vi "Test.vi"(10 "Test Controls":T8 {"Belts" scale=-1.0..1.0; "Arm" scale=-1.0..1.0; "Drive Train" scale=-1.0..1.0}, 11 "Call Context":T16) -> (0 "Loop 2 Data":T12, 1 "SubState 2":T11, 2 "Loop 1 Data":T13, 3 "SubState 1":T11, 4 "SubState 3":T11, 5 "Loop 0 Data":T14, 6 "Loop 3 Data":T10, 7 "SubState 0":T11=enum."driver control", 8 "SubState 4":T15, 9 "Test Data":T9)   [LabVIEW 2013]
uses:
  typedefs/State Machine/subStates.ctl
  <vilib>/Rock Robotics/WPI/DriverStation/WPI_DriverStationDerivedRobotMode.ctl
  typedefs/State Machine/singleUseSubstate.ctl
  typedefs/Loop Datatypes/Loop 0 Datatype.ctl
  typedefs/Loop Datatypes/Loop 1 Datatype.ctl
  typedefs/Loop Datatypes/Loop 2 Datatype.ctl
  typedefs/Loop Datatypes/Loop 3 Datatype.ctl
  typedefs/Test/test data.ctl
  typedefs/Test/test controls.ctl
  <vilib>/Rock Robotics/WPI/Compressor/WPI_CompressorDevRef.ctl
  <vilib>/Rock Robotics/WPI/DigitalInput/WPI_DigitalInputDevRef.ctl
  <vilib>/Rock Robotics/SystemInterfaces/DIO/FPGA_DIOChannel.ctl
  <vilib>/Rock Robotics/SystemInterfaces/Typedef/FPGA_TypedefDigitalModule.ctl
  <vilib>/Rock Robotics/WPI/Relay/WPI_RelayDevRef.ctl
  <vilib>/Rock Robotics/SystemInterfaces/DIO/FPGA_DIORelayChannel.ctl
  <vilib>/Rock Robotics/WPI/Relay/WPI_RelayDirection.ctl
  typedefs/fg_typedef.ctl
  typedefs/DevRef Type.ctl
  <vilib>/Rock Robotics/WPI/Solenoid/WPI_SolenoidGetEnum.vi
  <vilib>/Rock Robotics/WPI/Joystick/WPI_JoystickGetSetRefNum.vi
  <vilib>/Rock Robotics/WPI/Compressor/WPI_CompressorGetSetRefNum.vi
panel:
  out "CompressorDevRef":T1={"DevStatus"={"status"=FALSE, "code"=0, "source"=""}, "DigitalInputDevRef"={"DevStatus"={"status"=FALSE, "code"=0, "source"=""}, "DIO Channel"=enum."DIO 1", "Digital Module"=enum."Digital Module 1"}, "RelayDevRef"={"DevStatus"={"status"=FALSE, "code"=0, "source"=""}, "Relay Channel"=enum."Invalid", "Digital Module"=enum."Digital Module 1", "Relay Direction"=enum."Both directions"}}
  out "Compressor":bool
  out "JS Axis-Y 3":dbl
  out "JS Axis-X 3":dbl
  out "JS Axis-Y 2":dbl
  out "JS Axis-X 2":dbl
  out "UDB":bool
  out "JS Axis-X":dbl
  out "JS Axis-Y":dbl
  out "Exit Value":i32=-1
  # "Loop Data and Substates"
  # "Drive Loop"
  # "State Machine Master Loop"
  # "Pickup/Passing Belts Loop"
  # "Pickup/Passing Arm Loop"
  # "Pneumatics Loop"
  # "Test Code (Only Run in \nTest Mode)"
  # "Pneumatics"
  # "Home Encoders"
  # "Manual Override"
  # "Joystick Control"
  # "Arm Safeties"
  # "Drive Safeties"
  # "Sensors"
  # "Drive Encoders"
  # "Pneumatics Commands"
  # "Compressor"
  # "Arm Encoder"
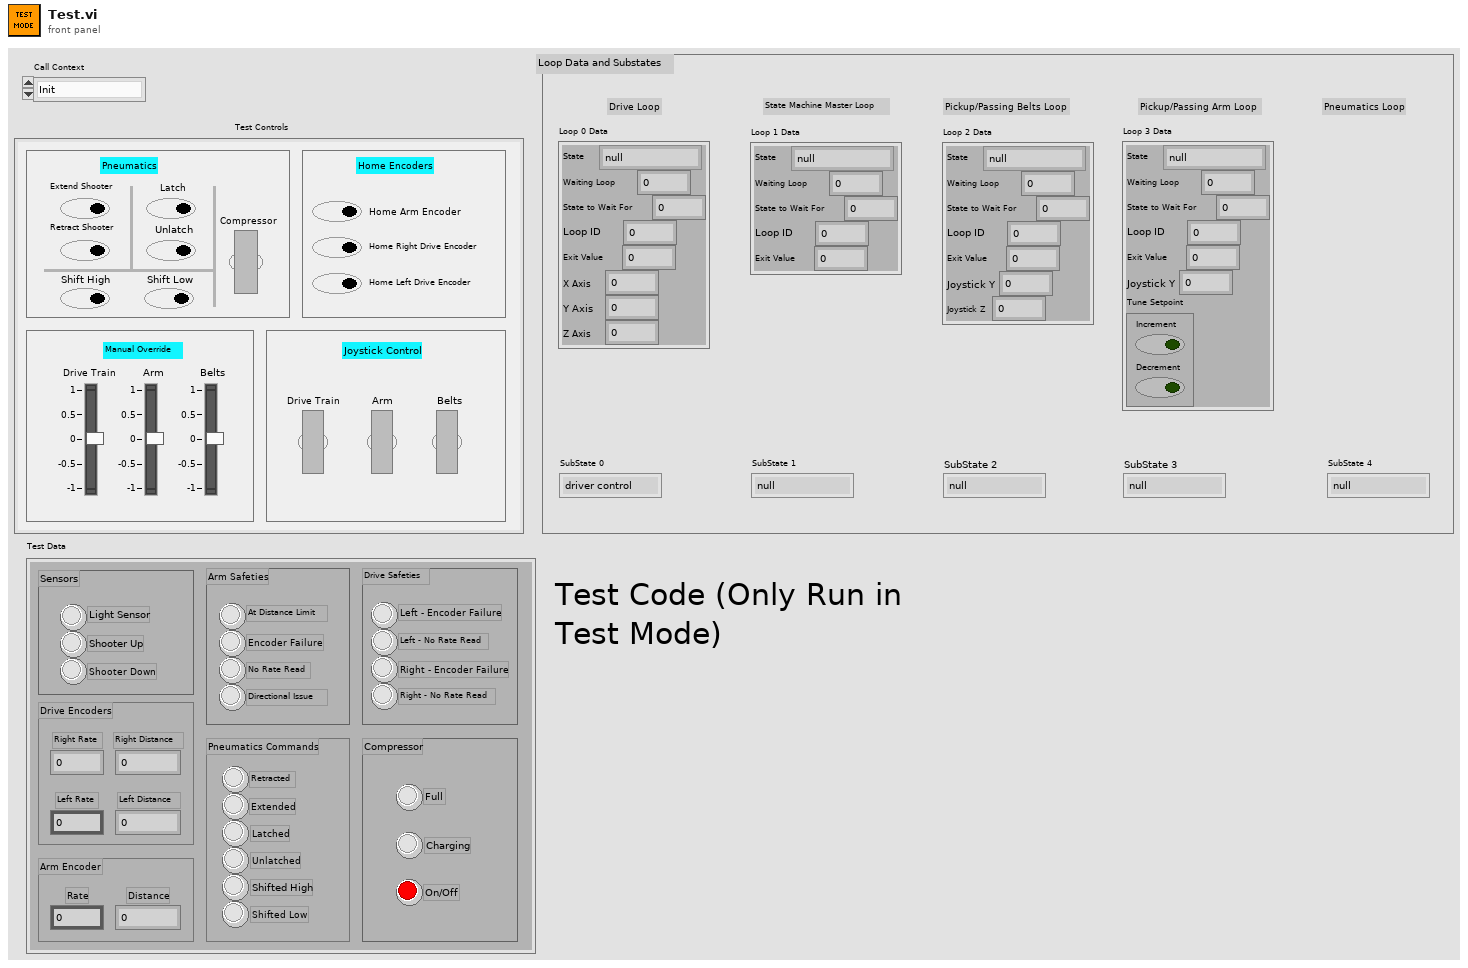
[diagram p1: front panel]
types:
  T1 = typedef "WPI_CompressorDevRef.ctl" = cluster{"DevStatus":errorcluster, "DigitalInputDevRef":T2, "RelayDevRef":T5}
  T2 = typedef "WPI_DigitalInputDevRef.ctl" = cluster{"DevStatus":errorcluster, "DIO Channel":T3, "Digital Module":T4}
  T3 = typedef "FPGA_DIOChannel.ctl" = enum8{"DIO 1", "DIO 2", "DIO 3", "DIO 4", "DIO 5", "DIO 6", "DIO 7", "DIO 8", "DIO 9", "DIO 10", "DIO 11", "DIO 12", "DIO 13", "DIO 14", "Invalid"}
  T4 = typedef "FPGA_TypedefDigitalModule.ctl" = enum16{"Digital Module 1", "Digital Module 2"}
  T5 = typedef "WPI_RelayDevRef.ctl" = cluster{"DevStatus":errorcluster, "Relay Channel":T6, "Digital Module":T4, "Relay Direction":T7}
  T6 = typedef "FPGA_DIORelayChannel.ctl" = enum8{"Relay 1", "Relay 2", "Relay 3", "Relay 4", "Relay 5", "Relay 6", "Relay 7", "Relay 8", "Invalid"}
  T7 = typedef "WPI_RelayDirection.ctl" = enum16{"Both directions", "Forward only", "Reverse only"}
  T8 = typedef "test controls.ctl" = cluster{"Drive Train":dbl, "Arm":dbl, "Belts":dbl, "Drive Train":bool, "Arm":bool, "Belts":bool, "Home Arm Encoder":bool, "Home Right Drive Encoder":bool, "Home Left Drive Encoder":bool, "Extend Shooter":bool, "Retract Shooter":bool, "Latch":bool, "Unlatch":bool, "Shift High":bool, "Shift Low":bool, "Compressor":bool}
  T9 = typedef "test data.ctl" = cluster{"Light Sensor":bool, "Shooter Up":bool, "Shooter Down":bool, "Left Rate":dbl, "Left Distance":dbl, "Right Rate":dbl, "Right Distance":dbl, "Rate":dbl, "Distance":dbl, "At Distance Limit":bool, "Encoder Failure":bool, "No Rate Read":bool, "Directional Issue":bool, "Latched":bool, "Unlatched":bool, "Shifted High":bool, "Shifted Low":bool, "Extended":bool, "Retracted":bool, "Left - Encoder Failure":bool, "Left - No Rate Read":bool, "Right - Encoder Failure":bool, "Right - No Rate Read":bool, "Charging":bool, "Full":bool, "On/Off":bool}
  T10 = typedef "Loop 3 Datatype.ctl" = cluster{"State":T11, "Waiting Loop":i32, "State to Wait For":i32, "Loop ID":i32, "Exit Value":i32, "Joystick Y":dbl, "Tune Setpoint":cluster{"Increment":bool, "Decrement":bool}}
  T11 = typedef "subStates.ctl" = enum16{"null", "wait", "driver control", "auto", "manual override", "hold position", "rotate", "pickup", "pass", "recover pass", "load", "goto shoot", "shoot high goal", "shoot low goal", "cancel arm", "cancel shooter", "end", "test"}
  T12 = typedef "Loop 2 Datatype.ctl" = cluster{"State":T11, "Waiting Loop":i32, "State to Wait For":i32, "Loop ID":i32, "Exit Value":i32, "Joystick Y":dbl, "Joystick Z":dbl}
  T13 = typedef "Loop 1 Datatype.ctl" = cluster{"State":T11, "Waiting Loop":i32, "State to Wait For":i32, "Loop ID":i32, "Exit Value":i32}
  T14 = typedef "Loop 0 Datatype.ctl" = cluster{"State":T11, "Waiting Loop":i32, "State to Wait For":i32, "Loop ID":i32, "Exit Value":i32, "X Axis":dbl, "Y Axis":dbl, "Z Axis":dbl}
  T15 = typedef "singleUseSubstate.ctl" = enum16{"null", "wait", "shift high", "shift low", "extend shooter", "retract shooter", "latch", "unlatch", "end"}
  T16 = typedef "WPI_DriverStationDerivedRobotMode.ctl" = enum16{"Init", "Execute", "Stop"}
  T17 = typedef "fg_typedef.ctl" = enum16{"Get", "Set"}
  T18 = typedef "DevRef Type.ctl" = enum16{"Shooter Solenoid", "Latch Solenoid", "Right Up Sensor", "Right Down Sensor", "Hold Sensor", "Arm Encoder"}
  T19 = typedef "WPI_EncoderDevRef.ctl" = cluster{"DevStatus":errorcluster, "EncoderIndex":T20, "CounterIndex":T21, "DistancePerCount":dbl, "Decoding Type":T22}
  T20 = typedef "FPGA_EncoderIdx.ctl" = enum8{"Enc 0", "Enc 1", "Enc 2", "Enc 3", "Invalid"}
  T21 = typedef "FPGA_CounterCtrSystemIndex.ctl" = enum8{"Ctr 0", "Ctr 1", "Ctr 2", "Ctr 3", "Ctr 4", "Ctr 5", "Ctr 6", "Ctr 7", "Invalid"}
  T22 = typedef "WPI_EncoderType.ctl" = enum16{"1x", "2x", "4x"}
  T23 = typedef "WPI_SolenoidDevRef.ctl" = cluster{"DevStatus":errorcluster, "Solenoid Module":T24, "Forward Solenoid Channel":T25, "Reverse Solenoid Channel":T25}
  T24 = typedef "FPGA_TypedefSolenoidModule.ctl" = enum16{"Solenoid Module 1", "Solenoid Module 2"}
  T25 = typedef "WPI_SolenoidChannel.ctl" = enum8{"Solenoid 1", "Solenoid 2", "Solenoid 3", "Solenoid 4", "Solenoid 5", "Solenoid 6", "Solenoid 7", "Solenoid 8", "Invalid"}
  T26 = typedef "WPI_JoystickDevRef.ctl" = cluster{"Device":T27}
  T27 = typedef "WPI_JoystickDeviceEnum.ctl" = enum16{"USB 1", "USB 2", "USB 3", "USB 4", "Kinect 1", "Kinect 2"}
  T28 = cluster{"axis 1 (x)":dbl, "axis 2 (y)":dbl, "axis 3 (throttle)":dbl, "axis 4":dbl, "axis 5":dbl, "axis 6":dbl}
  T29 = typedef "drive safety.ctl" = cluster{"Left - Encoder Failure":bool, "Left - No Rate Read":bool, "Right - Encoder Failure":bool, "Right - No Rate Read":bool}
  T30 = typedef "dashboard safety status data.ctl" = cluster{"At Distance Limit":bool, "No Rate Read":bool, "Encoder Failure":bool, "Encoder Directional Issue":bool}
  T31 = typedef "WPI_SolenoidValue.ctl" = enum16{"Off", "On", "Forward", "Reverse"}
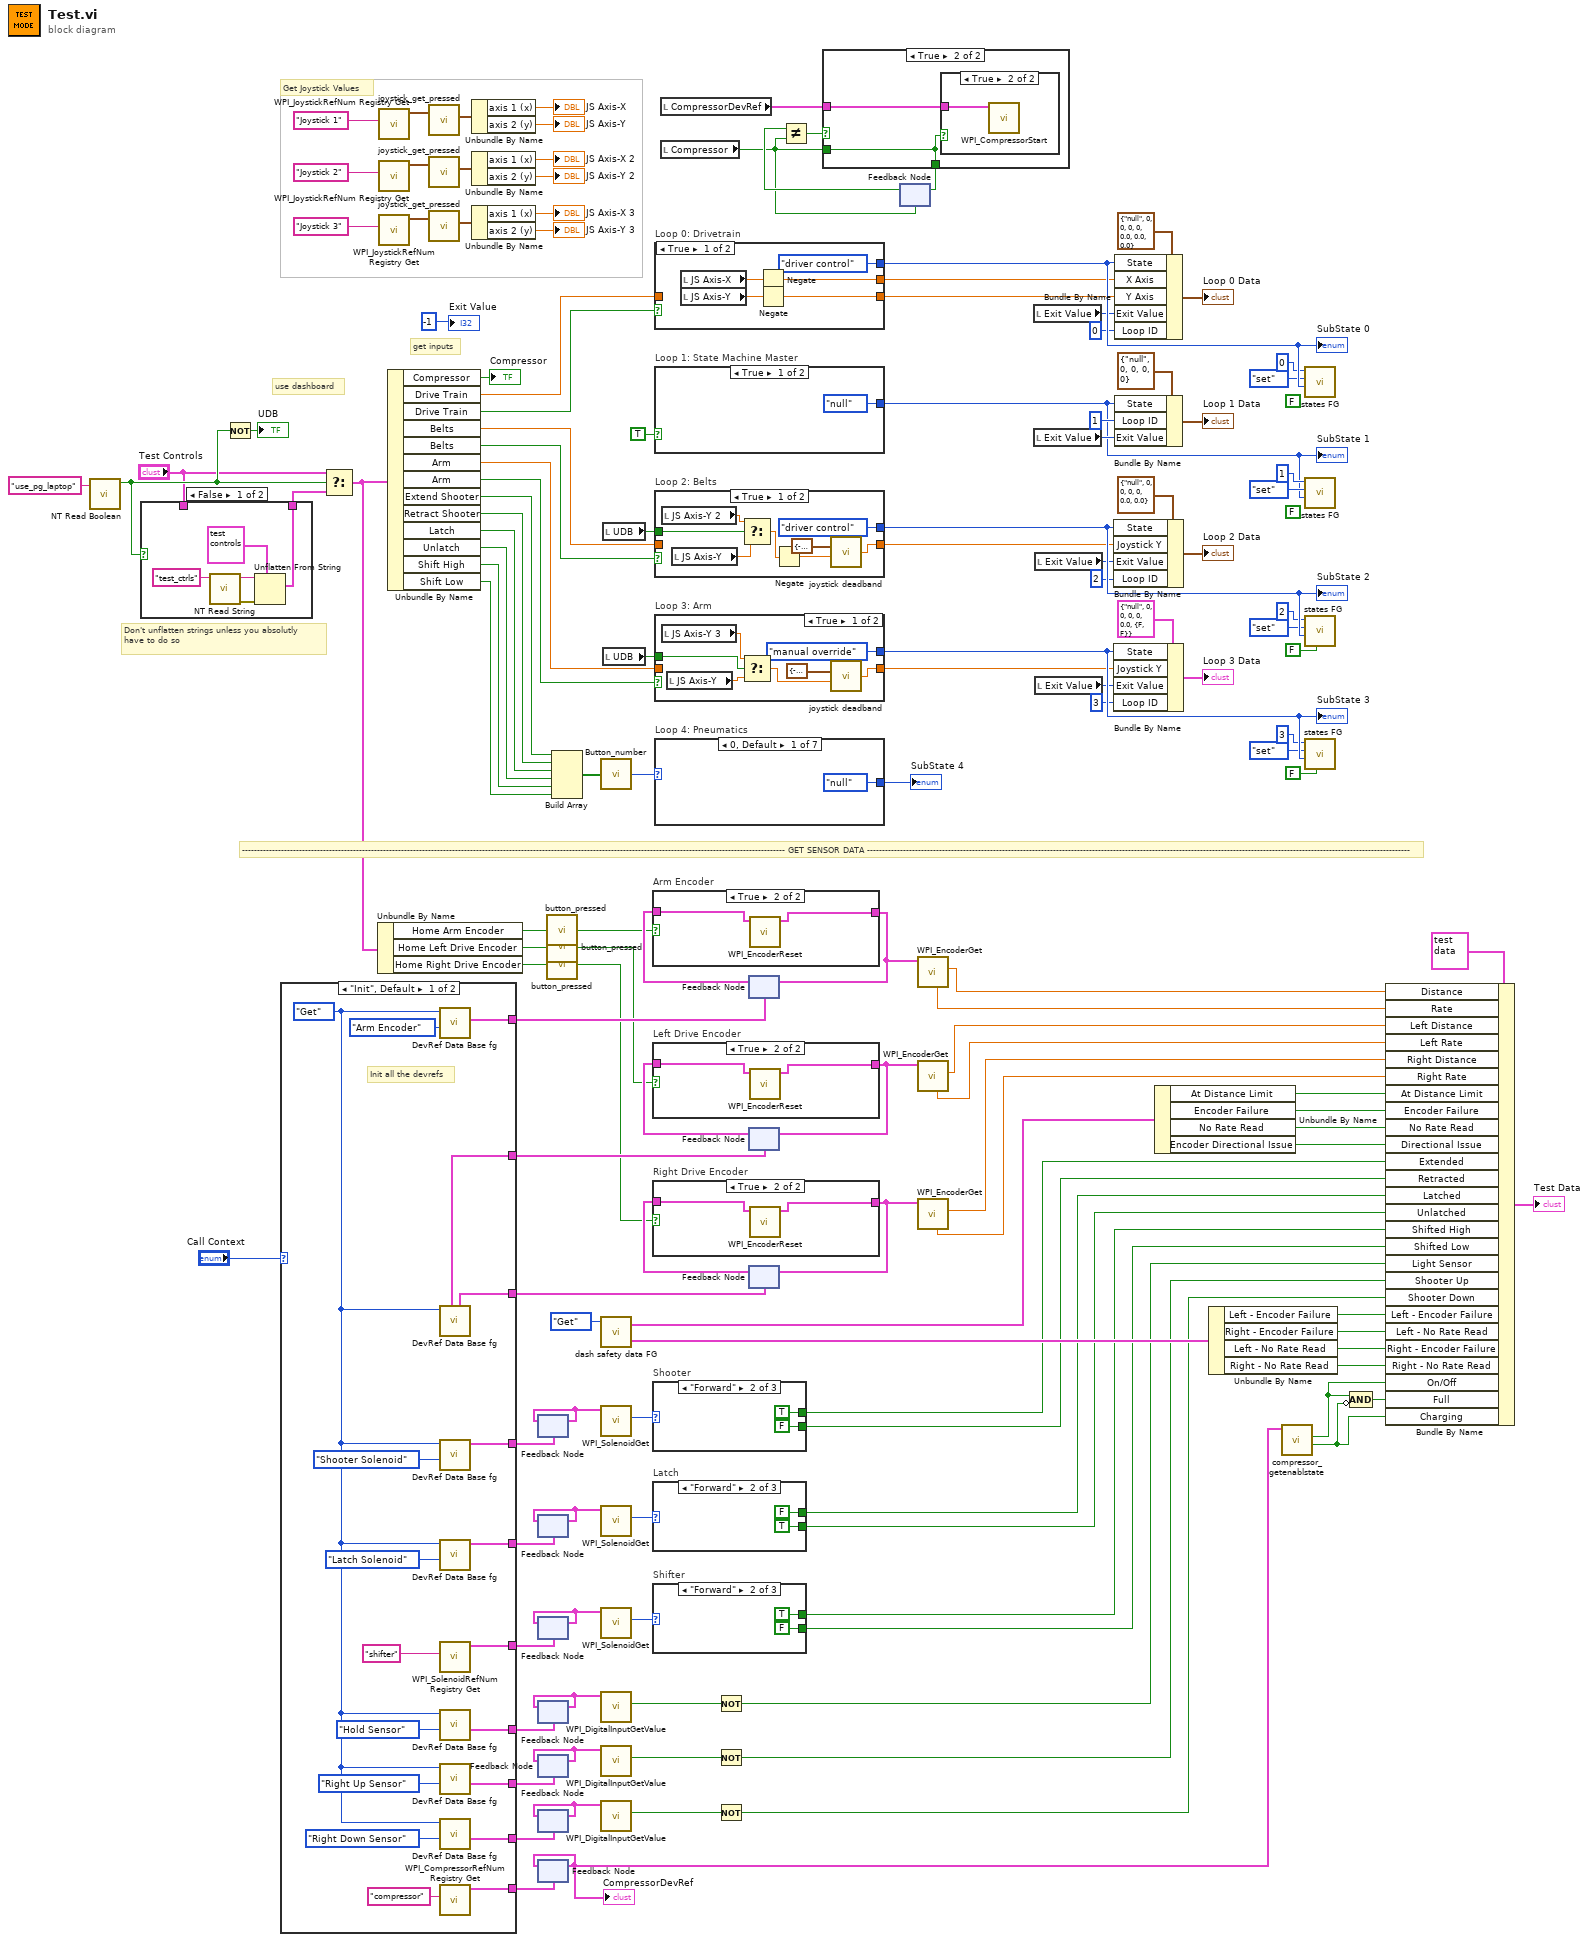
[diagram p0: block diagram]
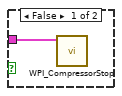
[diagram p3: hidden frame]
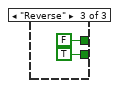
[diagram p6: hidden frame]
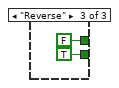
[diagram p8: hidden frame]
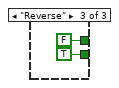
[diagram p10: hidden frame]
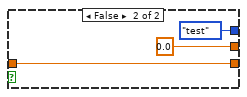
[diagram p15: hidden frame]
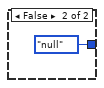
[diagram p16: hidden frame]
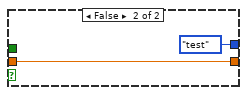
[diagram p17: hidden frame]
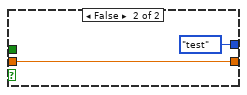
[diagram p18: hidden frame]
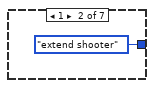
[diagram p19: hidden frame]
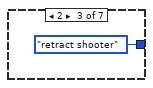
[diagram p20: hidden frame]
diagram:
  (unwired) FALSE ("exit in")
  (unwired) FALSE ("exit in")
  # "use dashboard"
  # "Don't unflatten strings unless you absolutly\nhave to do so"
  # "------------------------------------------------------------------------------------------------------------------------------------------------------------------------------------- GET SENSOR DATA -------------------------------------------------------------------------------------------------------------------------------------------------------------------------------------"
  # "get inputs"
  # "Get Joystick Values"
  n1 = call <vilib>:"NT Read Boolean.vi"("Name"="use_pg_laptop") -> ("Boolean"=w33:bool)  [unwired: 9 in, 1 out]
  n2 = case shown="False" w33 {
    tunnel: [w148 w153] -> w31
    tunnel: "Test Controls" -> [_ w153]
    frame False {
      n3 = call <vilib>:"NT Read String.vi"("Name"="test_ctrls") -> ("error out"=w151:errorcluster, "String"=w150:string)  [unwired: 9 in]
      n4 = Unflatten From String(type=T8 {"Drive Train"=0.0, "Arm"=0.0, "Belts"=0.0, "Drive Train"=FALSE, "Arm"=FALSE, "Belts"=FALSE, "Home Arm Encoder"=FALSE, "Home Right Drive Encoder"=FALSE, "Home Left Drive Encoder"=FALSE, "Extend Shooter"=FALSE, "Retract Shooter"=FALSE, "Latch"=FALSE, "Unlatch"=FALSE, "Shift High"=FALSE, "Shift Low"=FALSE, "Compressor"=FALSE} ("Test Controls"), binary string=w150, error in (no error)=w151) -> (value=w148:T8)  [unwired: 2 in, 2 out]
    }
    frame True {
    }
  }
  n5 = Not(x=w33) -> (.not. x?=→"UDB":bool)
  n6 = case shown="\"Init\", Default" "Call Context" {
    tunnel: [w171 _] -> w90
    tunnel: [w170 _] -> w86
    tunnel: [w169 _] -> w85
    tunnel: [w167 _] -> w63
    tunnel: [w166 _] -> w55
    tunnel: [w163 _] -> w52
    tunnel: [w161 _] -> w47
    tunnel: [w160 _] -> w42
    tunnel: [w157 _] -> w38
    tunnel: [w155 _] -> w12
    frame "Init", Default {
      w156 = fg_typedef."Get" ("Menu")
      # "Init all the devrefs"
      n7 = call "DevRef Data Base fg.vi"("DevRef to Get"=DevRef_Type."Arm Encoder", "Menu"=w156) -> ("Selected Encoder"=w171:T19)  [unwired: 1 in, 8 out]
      n8 = call "DevRef Data Base fg.vi"("Menu"=w156) -> ("right drive encoder"=w169:T19, "left drive encoder"=w170:T19)  [unwired: 2 in, 7 out]
      n9 = call "DevRef Data Base fg.vi"("DevRef to Get"=DevRef_Type."Shooter Solenoid", "Menu"=w156) -> ("Selected Solenoid"=w167:T23)  [unwired: 1 in, 8 out]
      n10 = call "DevRef Data Base fg.vi"("DevRef to Get"=DevRef_Type."Latch Solenoid", "Menu"=w156) -> ("Selected Solenoid"=w166:T23)  [unwired: 1 in, 8 out]
      n11 = call <vilib>:"WPI_SolenoidRefNum Registry Get.vi"("refnum name"="shifter") -> ("SolenoidDevRef"=w163:T23)  [unwired: 9 in, 1 out]
      n12 = call "DevRef Data Base fg.vi"("DevRef to Get"=DevRef_Type."Hold Sensor", "Menu"=w156) -> ("Selected Sensor"=w161:T2)  [unwired: 1 in, 8 out]
      n13 = call "DevRef Data Base fg.vi"("DevRef to Get"=DevRef_Type."Right Up Sensor", "Menu"=w156) -> ("Selected Sensor"=w160:T2)  [unwired: 1 in, 8 out]
      n14 = call "DevRef Data Base fg.vi"("DevRef to Get"=DevRef_Type."Right Down Sensor", "Menu"=w156) -> ("Selected Sensor"=w157:T2)  [unwired: 1 in, 8 out]
      n15 = call <vilib>:"WPI_CompressorRefNum Registry Get.vi"("refnum name"="compressor") -> ("CompressorDevRef"=w155:T1)  [unwired: 9 in, 1 out]
    }
    frame "Execute", "Stop" {
      # "do nothing"
    }
  }
  n16 = Select(t="Test Controls", s=w33, f=w31) -> (s? t:f=w34:T8)
  n17 = Unbundle By Name(w34) -> ("Home Arm Encoder"=w84:bool, "Home Left Drive Encoder"=w82:bool, "Home Right Drive Encoder"=w80:bool)
  n18 = call <vilib>:"WPI_JoystickRefNum Registry Get.vi"("refnum name"="Joystick 1") -> ("JoystickDevRef"=w133:T26)  [unwired: 9 in, 1 out]
  n19 = call <vilib>:"WPI_JoystickRefNum Registry Get.vi"("refnum name"="Joystick 2") -> ("JoystickDevRef"=w27:T26)  [unwired: 9 in, 1 out]
  n20 = call <vilib>:"WPI_JoystickRefNum Registry Get.vi"("refnum name"="Joystick 3") -> ("JoystickDevRef"=w24:T26)  [unwired: 9 in, 1 out]
  n21 = Unbundle By Name(w34) -> ("Compressor"=→"Compressor":bool, "Drive Train"=w105:dbl, "Drive Train"=w106:bool, "Belts"=w118:dbl, "Belts"=w119:bool, "Arm"=w137:dbl, "Arm"=w138:bool, "Extend Shooter"=w96:bool, "Retract Shooter"=w95:bool, "Latch"=w94:bool, "Unlatch"=w93:bool, "Shift High"=w92:bool, "Shift Low"=w91:bool)
  n22 = call "joystick_get_pressed.vi"("JoystickDevRef 2"=w133) -> ("Axes"=w131:T28)  [unwired: 1 in, 3 out]
  n23 = call "joystick_get_pressed.vi"("JoystickDevRef 2"=w27) -> ("Axes"=w28:T28)  [unwired: 1 in, 3 out]
  n24 = call "joystick_get_pressed.vi"("JoystickDevRef 2"=w24) -> ("Axes"=w23:T28)  [unwired: 1 in, 3 out]
  n25 = Unbundle By Name(w131) -> ("axis 1 (x)"=→"JS Axis-X":dbl, "axis 2 (y)"=→"JS Axis-Y":dbl)
  n26 = Unbundle By Name(w28) -> ("axis 1 (x)"=→"JS Axis-X 2":dbl, "axis 2 (y)"=→"JS Axis-Y 2":dbl)
  n27 = Unbundle By Name(w23) -> ("axis 1 (x)"=→"JS Axis-X 3":dbl, "axis 2 (y)"=→"JS Axis-Y 3":dbl)
  n28 = feedback #1(w63) -> (w61:T23)
  n29 = feedback-in #1(w61) -> ()
  n30 = feedback #2(w55) -> (w56:T23)
  n31 = feedback-in #2(w56) -> ()
  n32 = feedback #3(w52) -> (w51:T23)
  n33 = feedback-in #3(w51) -> ()
  n34 = feedback #4(w47) -> (w46:T2)
  n35 = feedback-in #4(w46) -> ()
  n36 = feedback #5(w42) -> (w43:T2)
  n37 = feedback-in #5(w43) -> ()
  n38 = feedback #6(w38) -> (w37:T2)
  n39 = feedback-in #6(w37) -> ()
  n40 = feedback #7(w12) -> (w1:T1)
  "CompressorDevRef" <- w1
  n41 = feedback-in #7(w1) -> ()
  n42 = call "button_pressed.vi"("Button In"=w84) -> ("Button Pressed?"=w83:bool)
  n43 = call "button_pressed.vi"("Button In"=w82) -> ("Button Pressed?"=w81:bool)
  n44 = call "button_pressed.vi"("Button In"=w80) -> ("Button Pressed?"=w79:bool)
  n45 = Build Array(w96, w95, w94, w93, w92, w91) -> (w143:bool[])
  n46 = call "Button_number.vi"("Button Array"=w143) -> ("Button Pressed"=w142:i32)
  n47 = call "dash safety data FG.vi"("Menu"=fg_typedef."Get") -> ("Drive Safety Data Out"=w147:T29, "Arm Safety Data Out"=w9:T30)  [unwired: 3 in]
  n48 = call-poly <vilib>:"WPI_SolenoidGet.vi"("SolenoidDevRef"=w61) -> ("Value"=w60:T31)  [unwired: 8 in, 2 out]
  n49 = call-poly <vilib>:"WPI_SolenoidGet.vi"("SolenoidDevRef"=w56) -> ("Value"=w57:T31)  [unwired: 8 in, 2 out]
  n50 = call-poly <vilib>:"WPI_SolenoidGet.vi"("SolenoidDevRef"=w51) -> ("Value"=w50:T31)  [unwired: 8 in, 2 out]
  n51 = call <vilib>:"WPI_DigitalInputGetValue.vi"("DigitalInputDevRef"=w46) -> ("Value"=w45:bool)  [unwired: 8 in, 2 out]
  n52 = call <vilib>:"WPI_DigitalInputGetValue.vi"("DigitalInputDevRef"=w43) -> ("Value"=w41:bool)  [unwired: 8 in, 2 out]
  n53 = call <vilib>:"WPI_DigitalInputGetValue.vi"("DigitalInputDevRef"=w37) -> ("Value"=w39:bool)  [unwired: 8 in, 2 out]
  n54 = local read "UDB"() -> (w19:bool)
  n55 = local read "UDB"() -> (w18:bool)
  n56 = case "Shooter" shown="\"Forward\"" w60 {
    tunnel: [_ TRUE FALSE] -> w59
    tunnel: [_ FALSE TRUE] -> w58
    frame "Off", Default {
    }
    frame "Forward" {
    }
    frame "Reverse" {
    }
  }
  n57 = case "Latch" shown="\"Forward\"" w57 {
    tunnel: [_ FALSE FALSE] -> w54
    tunnel: [_ TRUE TRUE] -> w53
    frame "Off", Default {
    }
    frame "Forward" {
    }
    frame "Reverse" {
    }
  }
  n58 = case "Shifter" shown="\"Forward\"" w50 {
    tunnel: [_ TRUE FALSE] -> w49
    tunnel: [_ FALSE TRUE] -> w48
    frame "Off", Default {
    }
    frame "Forward" {
    }
    frame "Reverse" {
    }
  }
  n59 = case "Loop 0: Drivetrain" shown="True" w106 {
    tunnel: w105 -> [_ w191]
    tunnel: [w185 w191] -> w97
    tunnel: [subStates."driver control" ("State") subStates."test" ("State")] -> w146
    tunnel: [w186 0.0 ("JS Axis-X")] -> w98
    frame True {
      n60 = local read "JS Axis-X"() -> (w188:dbl)
      n61 = local read "JS Axis-Y"() -> (w187:dbl)
      n62 = Negate(x=w188) -> (-x=w186:dbl)
      n63 = Negate(x=w187) -> (-x=w185:dbl)
    }
    frame False {
    }
  }
  "SubState 0" <- w146
  n64 = case "Loop 1: State Machine Master" shown="True" TRUE {
    tunnel: [subStates."null" ("State") subStates."null" ("State")] -> w107
    frame True {
    }
    frame False {
    }
  }
  "SubState 1" <- w107
  n65 = case "Loop 2: Belts" shown="True" w119 {
    tunnel: w118 -> [_ w203]
    tunnel: [w201 w203] -> w121
    tunnel: [subStates."driver control" ("State") subStates."test" ("State")] -> w145
    tunnel: w19 -> [w198 _]
    frame True {
      n66 = local read "JS Axis-Y 2"() -> (w195:dbl)
      n67 = local read "JS Axis-Y"() -> (w197:dbl)
      n68 = Select(t=w195, s=w198, f=w197) -> (s? t:f=w196:dbl)
      n69 = Negate(x=w196) -> (-x=w199:dbl)
      n70 = call "joystick deadband.vi"("Joystick In"=w199, "Deadband Range"=cluster{"Deadband Min":dbl, "Deadband Max":dbl} {"Deadband Min"=-0.09, "Deadband Max"=0.09}) -> ("Joystick Out"=w201:dbl)  [unwired: 4 in]
    }
    frame False {
    }
  }
  "SubState 2" <- w145
  n71 = case "Loop 3: Arm" shown="True" w138 {
    tunnel: w137 -> [_ w213]
    tunnel: [w210 w213] -> w135
    tunnel: [subStates."manual override" ("State") subStates."test" ("State")] -> w144
    tunnel: w18 -> [w205 _]
    frame True {
      n72 = local read "JS Axis-Y 3"() -> (w206:dbl)
      n73 = local read "JS Axis-Y"() -> (w208:dbl)
      n74 = Select(t=w206, s=w205, f=w208) -> (s? t:f=w207:dbl)
      n75 = call "joystick deadband.vi"("Joystick In"=w207, "Deadband Range"=cluster{"Deadband Min":dbl, "Deadband Max":dbl} {"Deadband Min"=-0.09, "Deadband Max"=0.09}) -> ("Joystick Out"=w210:dbl)  [unwired: 4 in]
    }
    frame False {
    }
  }
  "SubState 3" <- w144
  n76 = case "Loop 4: Pneumatics" shown="0, Default" w142 {
    tunnel: [singleUseSubstate."null" ("SubState 4") singleUseSubstate."extend shooter" ("SubState 4") singleUseSubstate."retract shooter" ("SubState 4") singleUseSubstate."latch" ("SubState 4") singleUseSubstate."unlatch" ("SubState 4") singleUseSubstate."shift high" ("SubState 4") singleUseSubstate."shift low" ("SubState 4")] -> w141
    frame 0, Default {
    }
    frame 1 {
    }
    frame 2 {
    }
    frame 3 {
    }
    frame 4 {
    }
    frame 5 {
    }
    frame 6 {
    }
  }
  "SubState 4" <- w141
  n77 = local read "CompressorDevRef"() -> (w11:T1)
  n78 = local read "Compressor"() -> (w13:bool)
  n79 = Not(x=w45) -> (.not. x?=w44:bool)
  n80 = Not(x=w41) -> (.not. x?=w40:bool)
  n81 = Not(x=w39) -> (.not. x?=w36:bool)
  n82 = feedback #8(w90) -> (w89:T19)
  n83 = case "Arm Encoder" shown="True" w83 {
    tunnel: w89 -> [w221 w223]
    tunnel: [w221 w222] -> w76
    frame False {
    }
    frame True {
      n84 = call <vilib>:"WPI_EncoderReset.vi"("EncoderDevRef"=w223) -> ("EncoderDevRef"=w222:T19)  [unwired: 9 in, 1 out]
    }
  }
  n85 = feedback-in #8(w76) -> ()
  n86 = feedback #9(w86) -> (w88:T19)
  n87 = case "Left Drive Encoder" shown="True" w81 {
    tunnel: w88 -> [w224 w226]
    tunnel: [w224 w225] -> w75
    frame False {
    }
    frame True {
      n88 = call <vilib>:"WPI_EncoderReset.vi"("EncoderDevRef"=w226) -> ("EncoderDevRef"=w225:T19)  [unwired: 9 in, 1 out]
    }
  }
  n89 = feedback-in #9(w75) -> ()
  n90 = feedback #10(w85) -> (w87:T19)
  n91 = case "Right Drive Encoder" shown="True" w79 {
    tunnel: w87 -> [w227 w229]
    tunnel: [w227 w228] -> w74
    frame False {
    }
    frame True {
      n92 = call <vilib>:"WPI_EncoderReset.vi"("EncoderDevRef"=w229) -> ("EncoderDevRef"=w228:T19)  [unwired: 9 in, 1 out]
    }
  }
  n93 = feedback-in #10(w74) -> ()
  n94 = feedback #11(w13) -> (w14:bool)
  n95 = Not Equal?(x=w14, y=w13) -> (x != y?=w15:bool)
  n96 = case shown="True" w15 {
    tunnel: w13 -> [w230 w232]
    tunnel: [w230 w232] -> w16
    tunnel: w11 -> [_ w231]
    frame False {
    }
    frame True {
      n97 = case shown="True" w232 {
        tunnel: w231 -> [w233 w234]
        frame False {
          n98 = call <vilib>:"WPI_CompressorStop.vi"("CompressorDevRef"=w233) -> ()  [unwired: 9 in, 2 out]
        }
        frame True {
          n99 = call <vilib>:"WPI_CompressorStart.vi"("CompressorDevRef"=w234) -> ()  [unwired: 9 in, 2 out]
        }
      }
    }
  }
  n100 = feedback-in #11(w16) -> ()
  n101 = call <vilib>:"WPI_EncoderGet.vi"("EncoderDevRef"=w76) -> ("Distance"=w73:dbl, "Rate"=w72:dbl)  [unwired: 5 in, 4 out]
  n102 = call <vilib>:"WPI_EncoderGet.vi"("EncoderDevRef"=w75) -> ("Distance"=w71:dbl, "Rate"=w70:dbl)  [unwired: 5 in, 4 out]
  n103 = call <vilib>:"WPI_EncoderGet.vi"("EncoderDevRef"=w74) -> ("Distance"=w69:dbl, "Rate"=w68:dbl)  [unwired: 5 in, 4 out]
  n104 = local read "Exit Value"() -> (w102:i32)
  n105 = local read "Exit Value"() -> (w115:i32)
  n106 = local read "Exit Value"() -> (w122:i32)
  n107 = local read "Exit Value"() -> (w132:i32)
  n108 = Bundle By Name(cluster=T12 {"State"=enum."null", "Waiting Loop"=0, "State to Wait For"=0, "Loop ID"=0, "Exit Value"=0, "Joystick Y"=0.0, "Joystick Z"=0.0} ("Loop 2 Data"), "State"=w145, "Joystick Y"=w121, "Exit Value"=w122, "Loop ID"=2) -> (→"Loop 2 Data":T12)
  n109 = Bundle By Name(cluster=T10 {"State"=enum."null", "Waiting Loop"=0, "State to Wait For"=0, "Loop ID"=0, "Exit Value"=0, "Joystick Y"=0.0, "Tune Setpoint"={"Increment"=FALSE, "Decrement"=FALSE}} ("Loop 3 Data"), "State"=w144, "Joystick Y"=w135, "Exit Value"=w132, "Loop ID"=3) -> (→"Loop 3 Data":T10)
  n110 = Bundle By Name(cluster=T14 {"State"=enum."null", "Waiting Loop"=0, "State to Wait For"=0, "Loop ID"=0, "Exit Value"=0, "X Axis"=0.0, "Y Axis"=0.0, "Z Axis"=0.0} ("Loop 0 Data"), "State"=w146, "X Axis"=w98, "Y Axis"=w97, "Exit Value"=w102, "Loop ID"=0) -> (→"Loop 0 Data":T14)
  n111 = Bundle By Name(cluster=T13 {"State"=enum."null", "Waiting Loop"=0, "State to Wait For"=0, "Loop ID"=0, "Exit Value"=0} ("Loop 1 Data"), "State"=w107, "Loop ID"=1, "Exit Value"=w115) -> (→"Loop 1 Data":T13)
  n112 = Unbundle By Name(w9) -> ("At Distance Limit"=w67:bool, "Encoder Failure"=w66:bool, "No Rate Read"=w65:bool, "Encoder Directional Issue"=w64:bool)
  n113 = Unbundle By Name(w147) -> ("Left - Encoder Failure"=w8:bool, "Right - Encoder Failure"=w7:bool, "Left - No Rate Read"=w6:bool, "Right - No Rate Read"=w5:bool)
  n114 = call "compressor_getenablstate.vi"("CompressorDevRef"=w1) -> ("Compressor Running"=w2:bool, "Enabled"=w4:bool)  [unwired: 7 in, 2 out]
  n115 = call "states FG.vi"("subState in"=w146, "menu (get)"=enum16{"set", "get"}."set", "Loop ID"=0) -> ()  [unwired: 5 in, 4 out]
  n116 = call "states FG.vi"("subState in"=w107, "menu (get)"=enum16{"set", "get"}."set", "Loop ID"=1) -> ()  [unwired: 5 in, 4 out]
  n117 = call "states FG.vi"("exit in"=FALSE, "subState in"=w145, "menu (get)"=enum16{"set", "get"}."set", "Loop ID"=2) -> ()  [unwired: 4 in, 4 out]
  n118 = call "states FG.vi"("exit in"=FALSE, "subState in"=w144, "menu (get)"=enum16{"set", "get"}."set", "Loop ID"=3) -> ()  [unwired: 4 in, 4 out]
  n119 = Compound Arithmetic op=AND(w4, invert w2) -> (w3:bool)
  n120 = Bundle By Name(cluster=T9 {"Light Sensor"=FALSE, "Shooter Up"=FALSE, "Shooter Down"=FALSE, "Left Rate"=0.0, "Left Distance"=0.0, "Right Rate"=0.0, "Right Distance"=0.0, "Rate"=0.0, "Distance"=0.0, "At Distance Limit"=FALSE, "Encoder Failure"=FALSE, "No Rate Read"=FALSE, "Directional Issue"=FALSE, "Latched"=FALSE, "Unlatched"=FALSE, "Shifted High"=FALSE, "Shifted Low"=FALSE, "Extended"=FALSE, "Retracted"=FALSE, "Left - Encoder Failure"=FALSE, "Left - No Rate Read"=FALSE, "Right - Encoder Failure"=FALSE, "Right - No Rate Read"=FALSE, "Charging"=FALSE, "Full"=FALSE, "On/Off"=FALSE} ("Test Data"), "Distance"=w73, "Rate"=w72, "Left Distance"=w71, "Left Rate"=w70, "Right Distance"=w69, "Right Rate"=w68, "At Distance Limit"=w67, "Encoder Failure"=w66, "No Rate Read"=w65, "Directional Issue"=w64, "Extended"=w59, "Retracted"=w58, "Latched"=w54, "Unlatched"=w53, "Shifted High"=w49, "Shifted Low"=w48, "Light Sensor"=w44, "Shooter Up"=w40, "Shooter Down"=w36, "Left - Encoder Failure"=w8, "Left - No Rate Read"=w7, "Right - Encoder Failure"=w6, "Right - No Rate Read"=w5, "On/Off"=w4, "Full"=w3, "Charging"=w2) -> (→"Test Data":T9)
  "Exit Value" <- -1 ("Exit Value")
